vi "WriteOnboardClockFrequency.vi"(8 "error in (no error)":errorcluster, 10 "Onboard clock frequency":dbl=100000000.0 format="%#_6p", 11 "FPGA VI Reference In":T1) -> (0 "error out":errorcluster, 3 "FPGA VI Reference Out":T1)   [LabVIEW 2012]
uses:
  Common FPGA VIs/Basic_FPGA_Ref.ctl
  <vilib>/Utility/error.llb/Error Cluster From Error Code.vi
  <vilib>/rvi/errors/niLvFpgaAdjustHostInterfaceError.vi
  <vilib>/rvi/interface/nirviReadWriteControl/nirviReadWriteControl.xnode
  <vilib>/rvi/interface/Simulation/niFpgaSimulationCallBeginRW.vi
  NiFpgaLv.dll
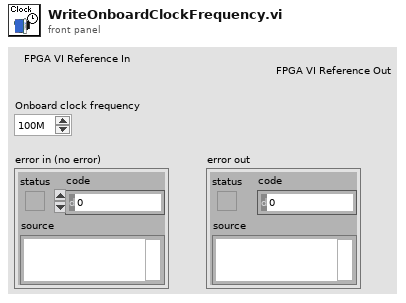
[diagram p1: front panel]
types:
  T1 = typedef "Basic_FPGA_Ref.ctl" = refnum<k20>
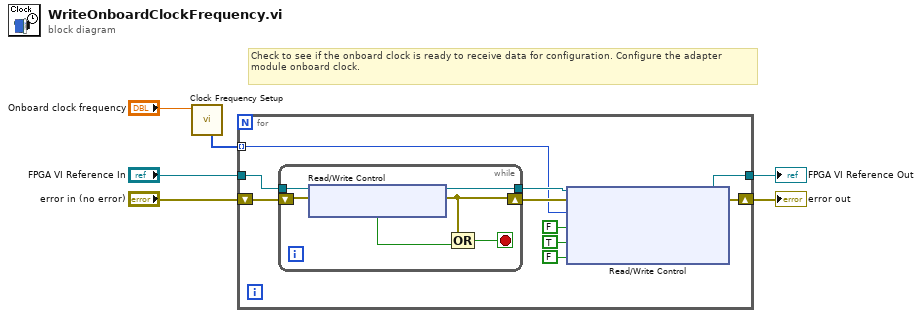
[diagram p0: block diagram]
diagram:
  # "Check to see if the onboard clock is ready to receive data for configuration. Configure the adapter module onboard clock."
  n1 = call "Clock Frequency Setup.vi"("Desired New Freq (Hz)"="Onboard clock frequency") -> ("Si570 Reg Address\nand Write Data"=w4:u16[])  [unwired: 6 in, 4 out]
  n2 = for {
    tunnel: "FPGA VI Reference In" -> [w7]
    shift-right: [w12] -> w5
    shift-left: "error in (no error)" -> [w16]
    tunnel: w4 -> [w13] mode=indexing
    tunnel: [w11] -> w1
    n3 = while {
      shift-right: [w19] -> w15
      shift-left: w16 -> [w22]
      tunnel: w7 -> [w21]
      tunnel: [w17] -> w14
      stop <- w20 stop-if-true
      n4 = xnode "Read/Write Control"("FPGA VI Reference In"=w21, "error in"=w22) -> ("FPGA VI Reference Out"=w17:T1, "error out"=w19:errorcluster, "Onboard_Clock_Ready"=w18:bool)
      n5 = Compound Arithmetic op=OR(w19, w18) -> (w20:bool)
    }
    n6 = xnode "Read/Write Control"("FPGA VI Reference In"=w14, "error in"=w15, "Onboard_Clock_Write_Data"=w13, "Onboard_Clock_Write"=FALSE, "Onboard_Clock_Write"=TRUE, "Onboard_Clock_Write"=FALSE) -> ("FPGA VI Reference Out"=w11:T1, "error out"=w12:errorcluster)
  }
  "error out" <- w5
  "FPGA VI Reference Out" <- w1
